vi "RPM to Pulse Width (Delay Time).vi"(4 "RPM":dbl) -> (0 "Period":dbl, 1 "Frequency":dbl, 2 "Low Time":dbl)   [LabVIEW 2019, in "SubVIs.lvlib" / "Tachometer VI.lvlib"]
uses:
  Tachometer VI.lvlib
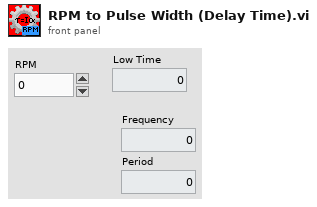
[diagram p1: front panel]
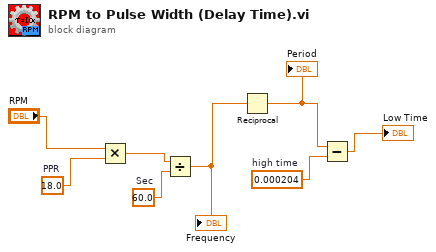
[diagram p0: block diagram]
diagram:
  w1 = 0.000204  # high time
  w2 = 18.0  # PPR
  w3 = 60.0  # Sec
  n1 = Multiply(x="RPM", y=w2) -> (x*y=w4:dbl)
  n2 = Divide(x=w4, y=w3) -> (x/y=w8:dbl)
  "Frequency" <- w8
  n3 = Reciprocal(x=w8) -> (1/x=w7:dbl)
  "Period" <- w7
  n4 = Subtract(x=w7, y=w1) -> (x-y=→"Low Time":dbl)
